vi "Day 11 Task 2.vi"() -> ()   [LabVIEW 2018]
panel:
  out "Step (part 2 answer)":i32
  # "Before any steps:\n11111\n19991\n19191\n19991\n11111\n\nAfter step 1:\n34543\n40004\n50005\n40004\n34543\n\nAfter step 2:\n45654\n51115\n61116\n51115\n45654"
  # "After step 1:\n6594254334\n3856965822\n6375667284\n7252447257\n7468496589\n5278635756\n3287952832\n7993992245\n5957959665\n6394862637"
  # "After step 2:\n8807476555\n5089087054\n8597889608\n8485769600\n8700908800\n6600088989\n6800005943\n0000007456\n9000000876\n8700006848"
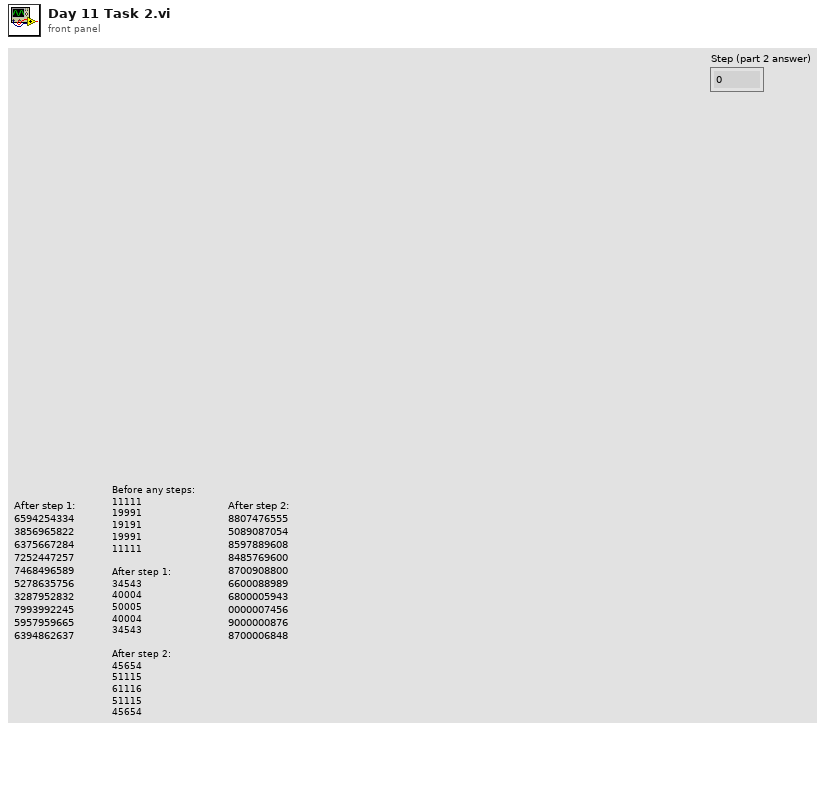
[diagram p1: front panel]
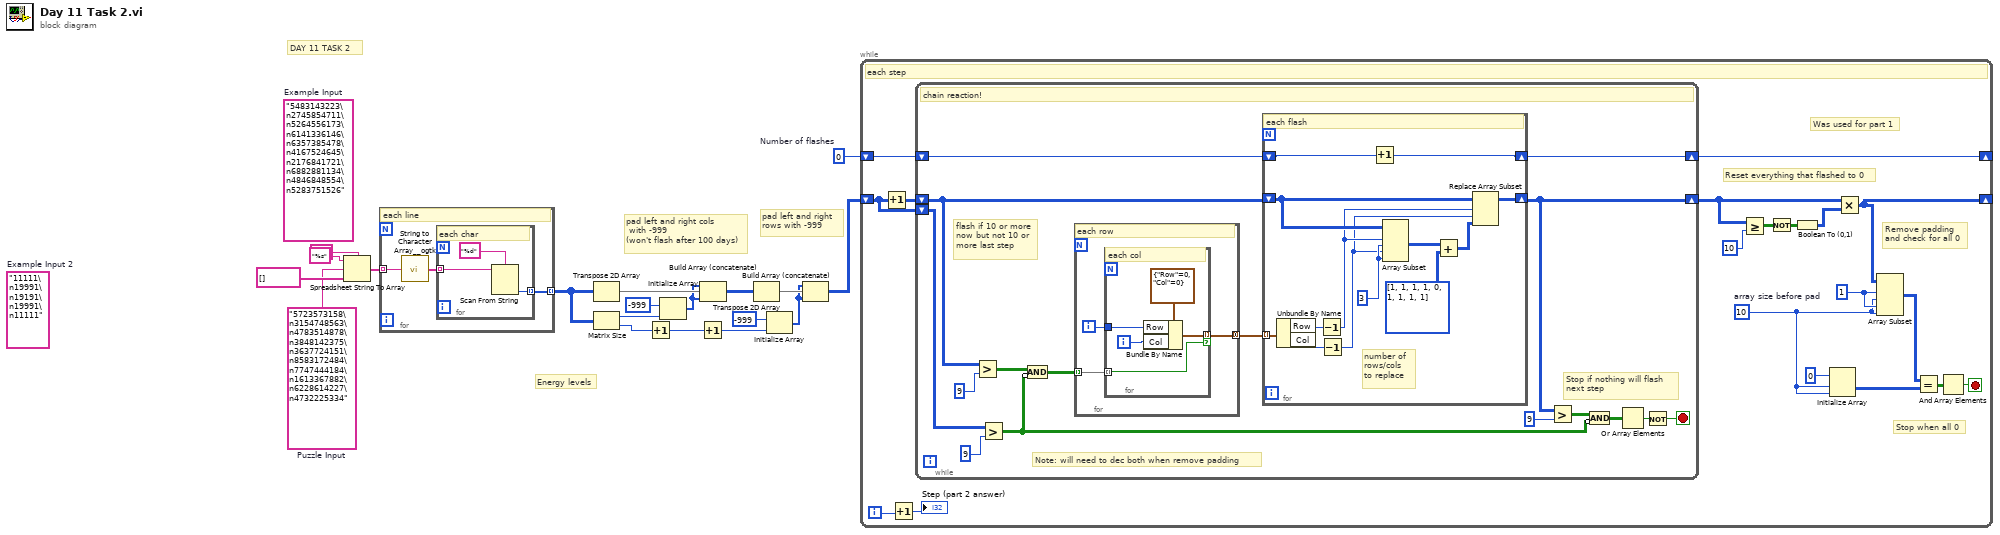
[diagram p0: block diagram]
diagram:
  w1 = "5723573158\n3154748563\n4783514878\n3848142375\n3637724151\n8583172484\n7747444184\n1613367882\n6228614227\n4732225334"  # Puzzle Input
  (unwired) "5483143223\n2745854711\n5264556173\n6141336146\n6357385478\n4167524645\n2176841721\n6882881134\n4846848554\n5283751526"  # Example Input
  w3 = 0  # Number of flashes
  (unwired) "11111\n19991\n19191\n19991\n11111"  # Example Input 2
  # "DAY 11 TASK 2"
  # "Energy levels"
  # "pad left and right \nrows with -999"
  # "pad left and right cols\n with -999 \n(won't flash after 100 days)"
  n1 = Spreadsheet String To Array(delimiter (Tab)="\n", format string="%s", spreadsheet string=w1, array type (2D Dbl)=string[] []) -> (array=w16:string[])
  n2 = for {
    tunnel: w16 -> [w22] mode=indexing
    tunnel: [w20] -> w4 mode=indexing
    # "each line"
    n3 = call <userlib>:"String to Character Array__ogtk.vi"("Input String"=w22) -> ("Character Array"=w21:string[])
    n4 = for {
      tunnel: w21 -> [w25] mode=indexing
      tunnel: [w23] -> w20 mode=indexing
      # "each char"
      n5 = Scan From String(format string="%d", input string=w25) -> (output 1=w23:i32)  [unwired: 3 in, 3 out]
    }
  }
  n6 = Transpose 2D Array(2D array=w4) -> (transposed array=w15:i32[][])
  n7 = Matrix Size(0:w4) -> (1:w11:i32, 2:w8:i32)
  n8 = Increment(x=w8) -> (x+1=w5:i32)
  n9 = Initialize Array(-999 ("element"), w11) -> (w10:i32[])
  n10 = Build Array (concatenate)(w10, w15, w10) -> (w14:i32[][])
  n11 = Increment(x=w5) -> (x+1=w7:i32)
  n12 = Transpose 2D Array(2D array=w14) -> (transposed array=w9:i32[][])
  n13 = Initialize Array(-999 ("number of columns"), w7) -> (w6:i32[])
  n14 = Build Array (concatenate)(w6, w9, w6) -> (w2:i32[][])
  n15 = while {
    shift-right: [w29] -> _
    shift-left: w2 -> [w36]
    shift-right: [w43] -> _
    shift-left: w3 -> [w44]
    i -> [w37]
    stop <- w30 stop-if-true
    w26 = 10  # array size before pad
    w28 = 1 ("index")
    # "Stop when all 0"
    # "Remove padding\nand check for all 0"
    # "Was used for part 1"
    # "Reset everything that flashed to 0"
    # "each step"
    n16 = Increment(x=w36) -> (x+1=w38:i32[][])
    n17 = Increment(x=w37) -> (x+1=→"Step (part 2 answer)":i32)
    n18 = while {
      shift-right: [w57] -> w43
      shift-left: w44 -> [w58]
      shift-right: [w50] -> w34
      shift-left: w38 -> [w49]
      shift-left: w36 -> [w48]
      stop <- w45 stop-if-true
      # "flash if 10 or more\nnow but not 10 or\nmore last step"
      # "Stop if nothing will flash \nnext step"
      # "Note: will need to dec both when remove padding"
      # "chain reaction!"
      n19 = Greater?(x=w49, y=9) -> (0:w55:bool[][])
      n20 = Greater?(x=w48, y=9) -> (0:w52:bool[][])
      n21 = Compound Arithmetic op=AND(w55, invert w52) -> (w47:bool[][])
      n22 = for {
        tunnel: w47 -> [w76] mode=indexing
        tunnel: [w74] -> w59 mode=concatenating
        i -> [w75]
        # "each row"
        n23 = for {
          tunnel: w76 -> [w79] mode=indexing
          tunnel: w75 -> [w77]
          tunnel: [w80] -> w74 mode=indexing if=w79
          i -> [w78]
          # "each col"
          n24 = Bundle By Name(cluster=cluster{"Row":i32, "Col":i32} {"Row"=0, "Col"=0}, "Row"=w77, "Col"=w78) -> (w80:cluster{"Row":i32, "Col":i32})
        }
      }
      n25 = for {
        tunnel: w59 -> [w73] mode=indexing
        shift-right: [w68] -> w50
        shift-left: w49 -> [w69]
        shift-right: [w67] -> w57
        shift-left: w58 -> [w66]
        w72 = 3 ("length")
        # "number of \nrows/cols\nto replace"
        # "each flash"
        n26 = Unbundle By Name(w73) -> ("Row"=w65:i32, "Col"=w64:i32)
        n27 = Decrement(x=w65) -> (x-1=w63:i32)
        n28 = Decrement(x=w64) -> (x-1=w62:i32)
        n29 = Increment(x=w66) -> (x+1=w67:i32)
        n30 = Array Subset(array=w69, index (row)=w63, length (row)=w72, index (col)=w62, length (col)=w72) -> (w71:i32[][])
        n31 = Add(x=w71, y=i32[][] [[1, 1, 1], [1, 0, 1], [1, 1, 1]]) -> (x+y=w61:i32[][])
        n32 = Replace Array Subset(array=w69, new element=w61, index (row)=w63, index (col)=w62) -> (w68:i32[][])
      }
      n33 = Greater?(x=w50, y=9) -> (0:w53:bool[][])
      n34 = Compound Arithmetic op=AND(w53, invert w52) -> (w51:bool[][])
      n35 = Or Array Elements(Boolean array=w51) -> (logical OR=w46:bool)
      n36 = Not(x=w46) -> (.not. x?=w45:bool)
    }
    n37 = Greater Or Equal?(x=w34, y=10) -> (x >= y?=w41:bool[][])
    n38 = Not(x=w41) -> (.not. x?=w40:bool[][])
    n39 = Boolean To (0,1)(Boolean=w40) -> (0, 1=w39:i16[][])
    n40 = Initialize Array(0, w26, w26) -> (w32:i32[][])
    n41 = Multiply(x=w34, y=w39) -> (x*y=w29:i32[][])
    n42 = Array Subset(array=w29, index (row)=w28, length (row)=w26, index (col)=w28, length (col)=w26) -> (w27:i32[][])
    n43 = Equal?(x=w27, y=w32) -> (x = y?=w31:bool[][])
    n44 = And Array Elements(Boolean array=w31) -> (logical AND=w30:bool)
  }
